vi "NI-USB-6210_Kernel.vi"() -> (0 "error out":errorcluster)   [LabVIEW 2013]
uses:
  <vilib>/DAQmx/read.llb/DAQmx Read (Analog 2D DBL NChan NSamp).vi
  Globals/measurementGlobal.vi
  <vilib>/DAQmx/configure/timing.llb/DAQmx Timing (Sample Clock).vi
  <vilib>/DAQmx/create/channels.llb/DAQmx Create Channel (AI-Voltage-Basic).vi
  <vilib>/DAQmx/miscellaneous.llb/DAQmx Fill In Error Info.vi
panel:
  out "Block Index":i32
  out "Case":string[](array[string])
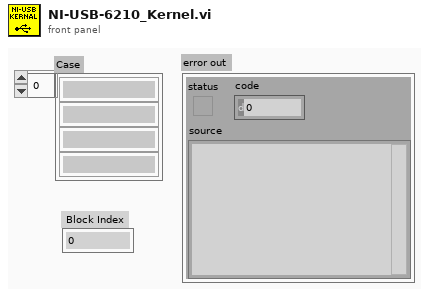
[diagram p1: front panel]
types:
  T1 = cluster{"No of Chans":i32, "Low Volt Limit (-10V)":dbl, "High Volt Limit (10V)":dbl}[]
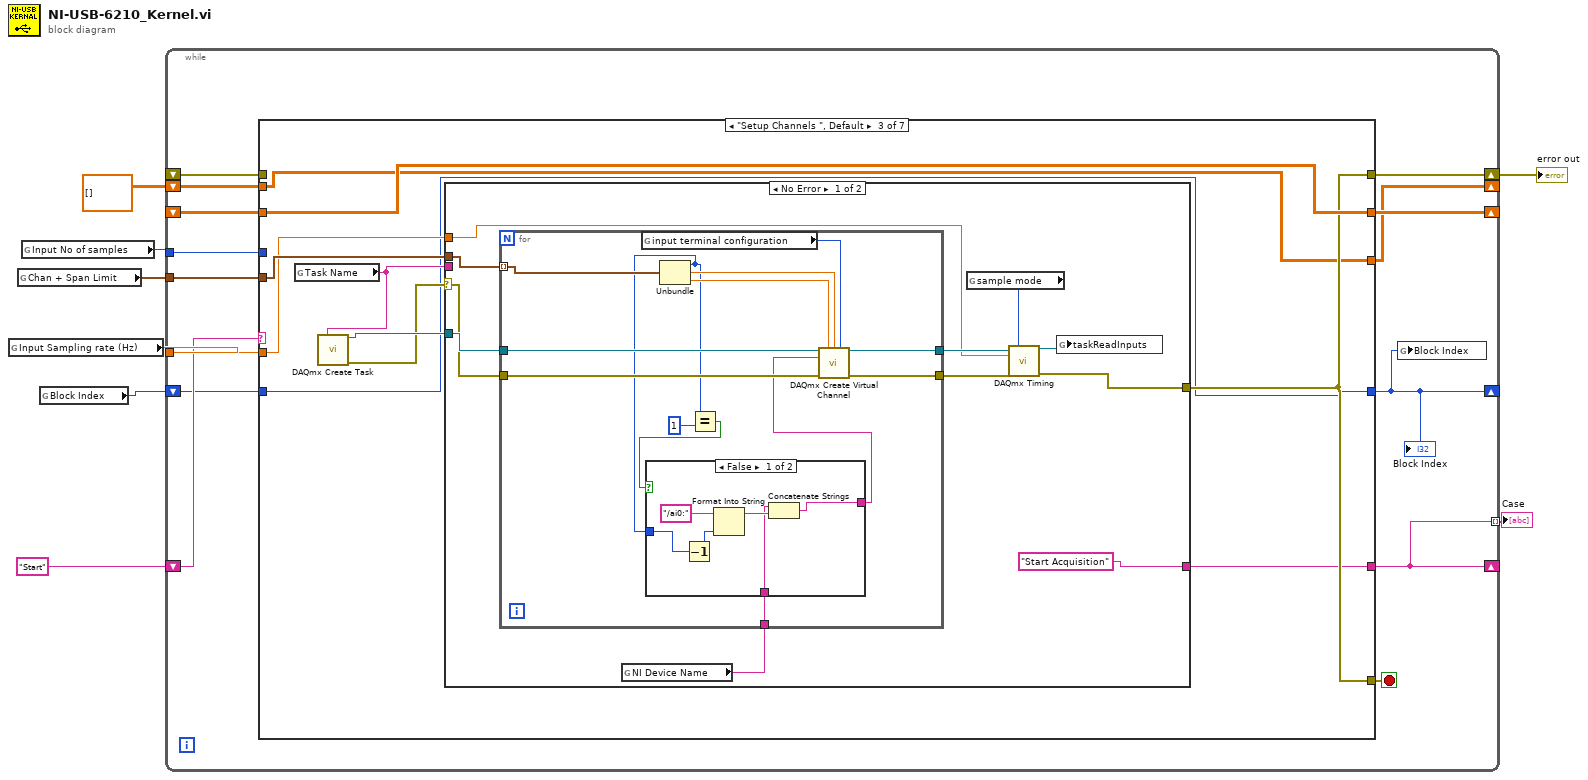
[diagram p0: block diagram]
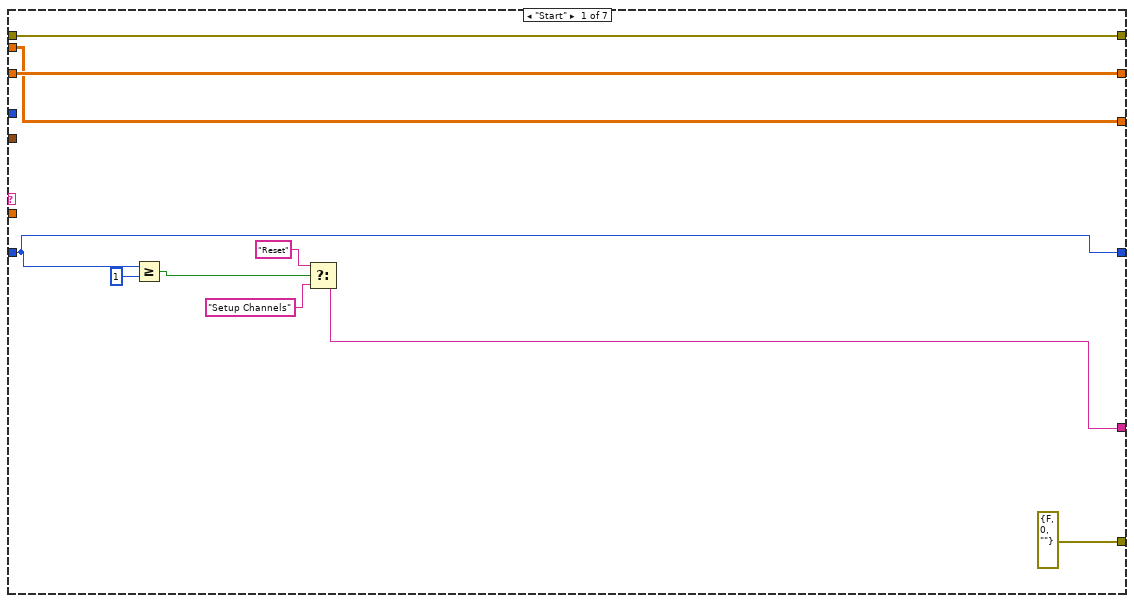
[diagram p2: hidden frame]
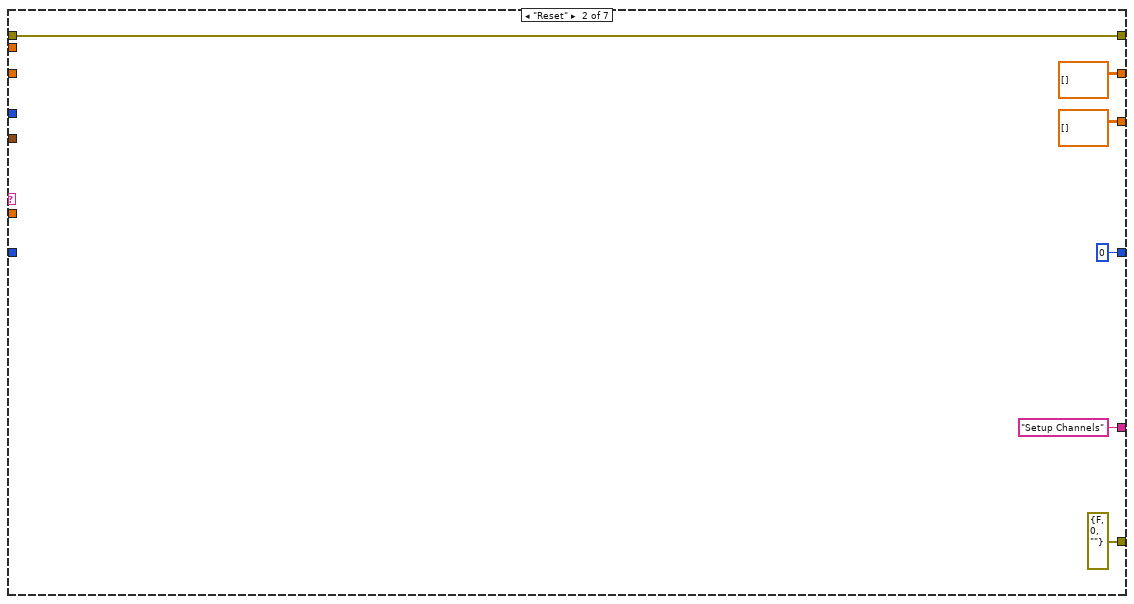
[diagram p3: hidden frame]
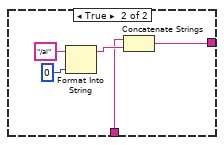
[diagram p4: hidden frame]
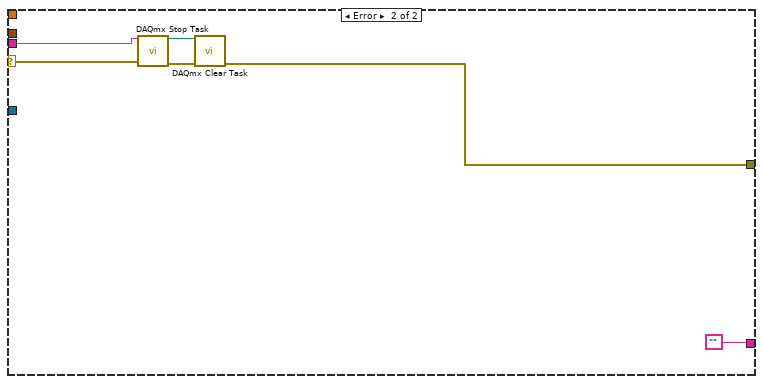
[diagram p5: hidden frame]
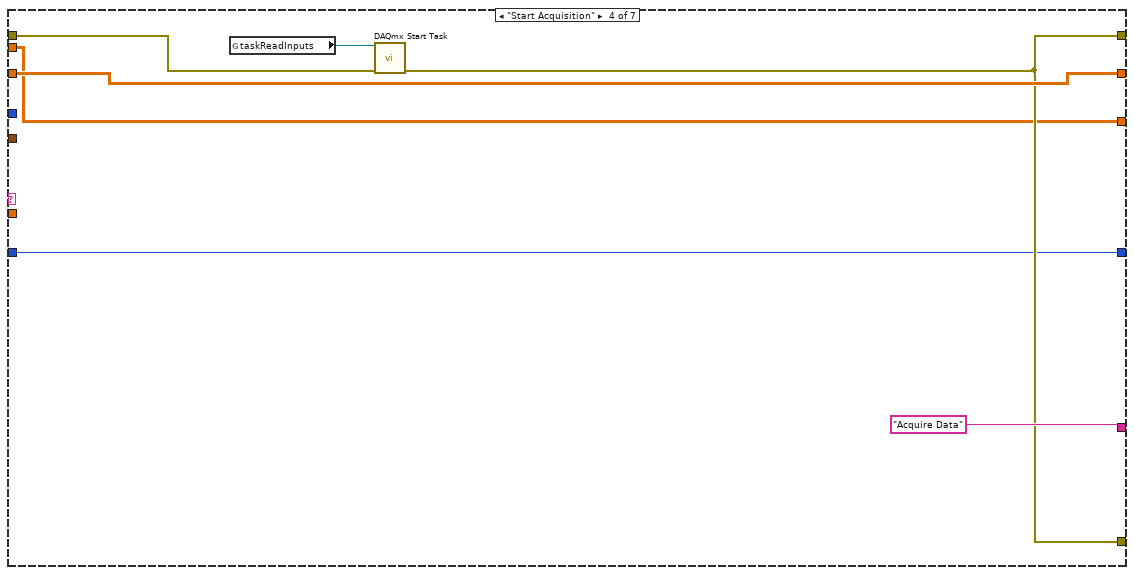
[diagram p6: hidden frame]
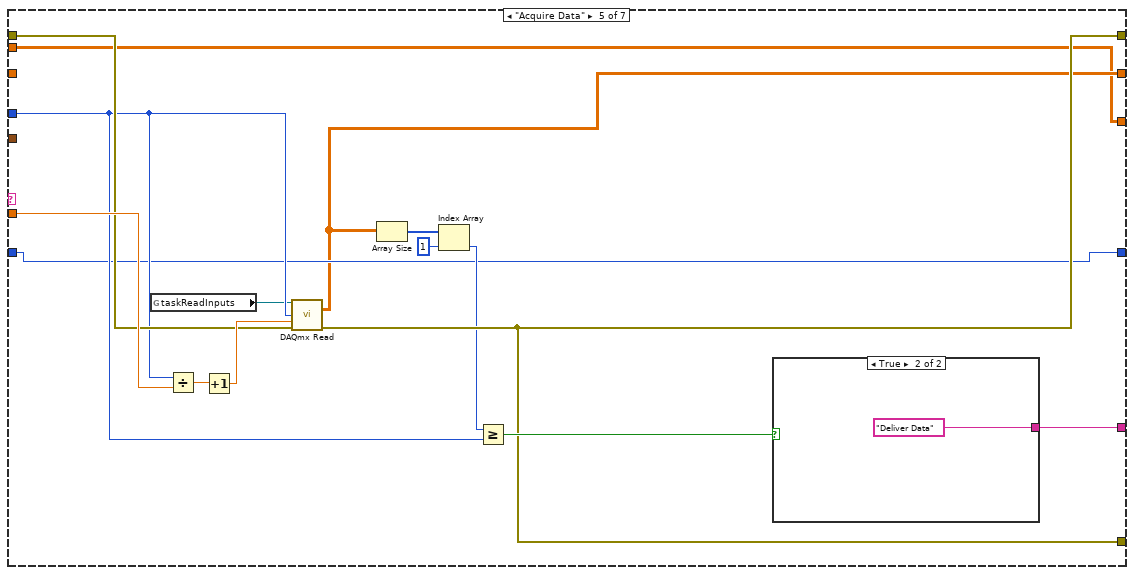
[diagram p7: hidden frame]
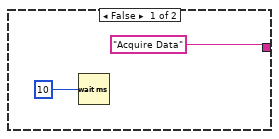
[diagram p8: hidden frame]
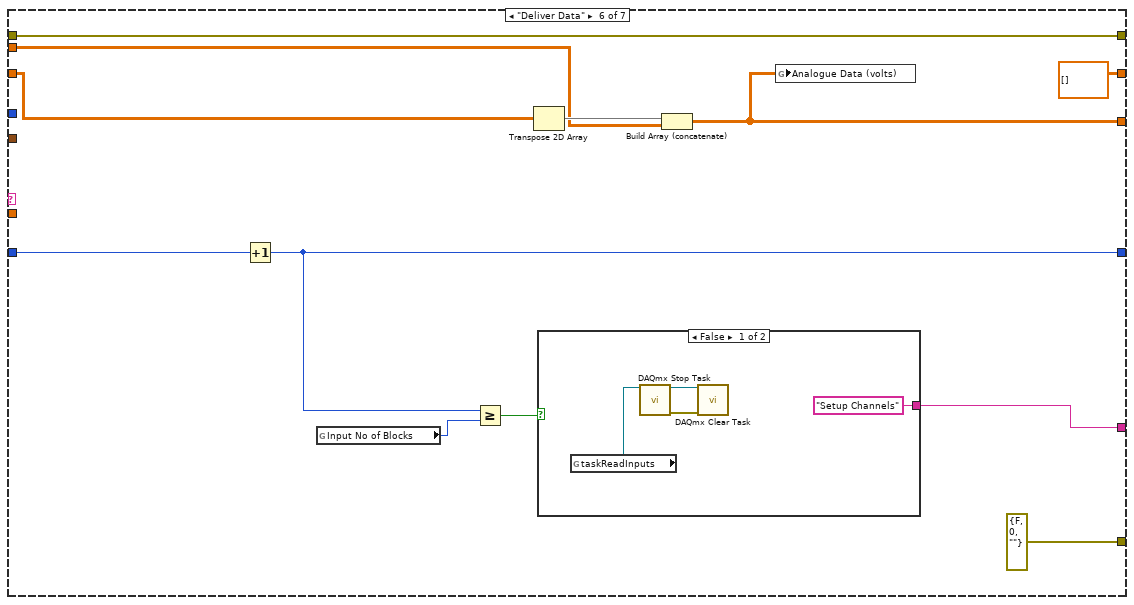
[diagram p9: hidden frame]
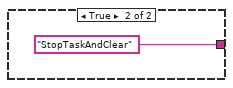
[diagram p10: hidden frame]
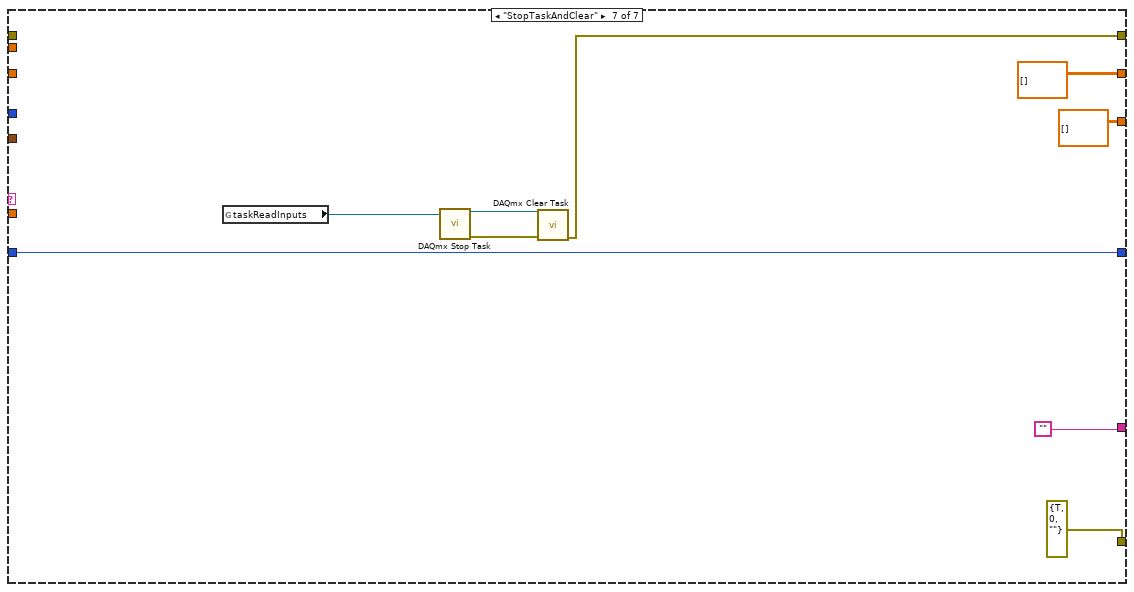
[diagram p11: hidden frame]
diagram:
  n1 = global read "measurementGlobal.vi" "Input Sampling rate (Hz)"() -> (w7:dbl)
  n2 = global read "measurementGlobal.vi" "Chan + Span Limit"() -> (w3:T1)
  n3 = global read "measurementGlobal.vi" "Input No of samples"() -> (w8:i32)
  n4 = global read "measurementGlobal.vi" "Block Index"() -> (w2:i32)
  n5 = while {
    tunnel: w8 -> [w22]
    tunnel: w7 -> [w21]
    shift-right: [w20] -> w6
    shift-left: _ -> [w19]
    shift-right: [w10] -> _
    shift-left: _ -> [w17]
    shift-right: [w15] -> _
    shift-left: "Start" -> [w16]
    tunnel: [w15] -> w4 mode=indexing
    tunnel: w3 -> [w14]
    shift-right: [w12] -> _
    shift-left: w2 -> [w13]
    shift-right: [w9] -> _
    shift-left: dbl[][] [] ("data") -> [w11]
    stop <- w18 stop-if-true
    n6 = case shown="\"Setup Channels \", Default" w16 {
      tunnel: w22 -> [_ _ _ _ w105 _ _]
      tunnel: w21 -> [_ _ w43 _ w111 _ _]
      tunnel: [w25 w35 w42 w92 w102 w126 w138] -> w20
      tunnel: w19 -> [w25 w35 _ w95 w108 w126 _]
      tunnel: [errorcluster {"status"=FALSE, "code"=0, "source"=""} ("error out") errorcluster {"status"=FALSE, "code"=0, "source"=""} ("error out") w42 w92 w102 errorcluster {"status"=FALSE, "code"=0, "source"=""} ("error out") errorcluster {"status"=TRUE, "code"=0, "source"=""} ("error out")] -> w18
      tunnel: [w32 dbl[][] [] ("data") w48 w94 w98 dbl[][] [] ("data") dbl[][] [] ("data")] -> w10
      tunnel: w17 -> [w32 _ w48 w94 _ w118 _]
      tunnel: [w27 "Setup Channels" ("f") w41 "Acquire Data" w103 w123 ""] -> w15
      tunnel: w14 -> [_ _ w44 _ _ _ _]
      tunnel: w13 -> [w26 _ w40 w91 w99 w120 w133]
      tunnel: [w26 0 ("Block Index") w40 w91 w99 w119 w133] -> w12
      tunnel: w11 -> [w23 _ w39 w90 w97 w116 _]
      tunnel: [w23 dbl[][] [] ("data") w39 w90 w97 w115 dbl[][] [] ("data")] -> w9
      frame "Start" {
        n7 = Greater Or Equal?(x=w26, y=1) -> (x >= y?=w30:bool)
        n8 = Select(t="Reset", s=w30, f="Setup Channels") -> (s? t:f=w27:string)
      }
      frame "Reset" {
      }
      frame "Setup Channels ", Default {
        n9 = global read "measurementGlobal.vi" "Task Name"() -> (w45:string)
        n10 = call <vilib>:"DAQmx Create Task.vi"("new task name"=w45) -> ("task out"=w47:refnum<k21>, "error out"=w46:errorcluster)  [unwired: 13 in]
        n11 = case shown="No Error" w46 {
          selector: w46 -> [w57 w86]
          tunnel: w44 -> [w56 _]
          tunnel: w47 -> [w58 _]
          tunnel: w45 -> [_ w88]
          tunnel: [w50 w85] -> w42
          tunnel: w43 -> [w52 _]
          tunnel: ["Start Acquisition" ""] -> w41
          frame No Error {
            n12 = global read "measurementGlobal.vi" "NI Device Name"() -> (w59:string)
            n13 = for {
              tunnel: w56 -> [w72] mode=indexing
              tunnel: w59 -> [w62]
              tunnel: [w69] -> w53
              tunnel: [w68] -> w51
              tunnel: w58 -> [w66]
              tunnel: w57 -> [w65]
              n14 = global read "measurementGlobal.vi" "input terminal configuration"() -> (w67:i32)
              n15 = Unbundle(w72) -> ("No of Chans"=w61:i32, "Low Volt Limit (-10V)"=w71:dbl, "High Volt Limit (10V)"=w70:dbl)
              n16 = Equal?(x=w61, y=1) -> (x = y?=w63:bool)
              n17 = case shown="False" w63 {
                tunnel: w62 -> [w73 w81]
                tunnel: [w76 w80] -> w60
                tunnel: w61 -> [w75 _]
                frame False {
                  n18 = Decrement(x=w75) -> (x-1=w74:i32)
                  n19 = Format Into String(initial string="/ai0:", w74) -> (resulting string=w78:string)  [unwired: 2 in, 1 out]
                  n20 = Concatenate Strings(w73, w78) -> (w76:string)
                }
                frame True {
                  n21 = Format Into String(initial string="/ai", 0 ("input 1")) -> (resulting string=w82:string)  [unwired: 2 in, 1 out]
                  n22 = Concatenate Strings(w81, w82) -> (w80:string)
                }
              }
              n23 = call-poly <vilib>:"DAQmx Create Virtual Channel.vi"("task in"=w66, "maximum value"=w70, "minimum value"=w71, "input terminal configuration"=w67, "physical channels"=w60, "error in"=w65) -> ("task out"=w69:refnum<k21>, "error out"=w68:errorcluster)  [unwired: 8 in]
            }
            n24 = global read "measurementGlobal.vi" "sample mode"() -> (w55:i32)
            n25 = call-poly <vilib>:"DAQmx Timing.vi"("task/channels in"=w53, "sample mode"=w55, "rate"=w52, "error in"=w51) -> ("task out"=w54:refnum<k21>, "error out"=w50:errorcluster)  [unwired: 10 in]
            n26 = global write "measurementGlobal.vi" "taskReadInputs"(w54) -> ()
          }
          frame Error {
            n27 = call <vilib>:"DAQmx Stop Task.vi"("task/channels in"=w88, "error in"=w86) -> ("task out"=w87:refnum<k21>, "error out"=w89:errorcluster)  [unwired: 12 in]
            n28 = call <vilib>:"DAQmx Clear Task.vi"("task in"=w87, "error in"=w89) -> ("error out"=w85:errorcluster)  [unwired: 13 in]
          }
        }
      }
      frame "Start Acquisition" {
        n29 = global read "measurementGlobal.vi" "taskReadInputs"() -> (w96:refnum<k21>)
        n30 = call <vilib>:"DAQmx Start Task.vi"("task/channels in"=w96, "error in"=w95) -> ("error out"=w92:errorcluster)  [unwired: 12 in, 1 out]
      }
      frame "Acquire Data" {
        n31 = global read "measurementGlobal.vi" "taskReadInputs"() -> (w101:refnum<k21>)
        n32 = Divide(x=w105, y=w111) -> (x/y=w110:dbl)
        n33 = Increment(x=w110) -> (x+1=w109:dbl)
        n34 = call-poly <vilib>:"DAQmx Read.vi"("task/channels in"=w101, "number of samples per channel"=w105, "timeout"=w109, "error in"=w108) -> ("data"=w98:dbl[][], "error out"=w102:errorcluster)  [unwired: 9 in, 1 out]
        n35 = Array Size(array=w98) -> (size(s)=w107:i32[])
        n36 = Index Array(array=w107, index=1) -> (element=w100:i32)
        n37 = Greater Or Equal?(x=w100, y=w105) -> (x >= y?=w104:bool)
        n38 = case shown="True" w104 {
          tunnel: ["Acquire Data" "Deliver Data"] -> w103
          frame False {
            n39 = Wait (ms)(milliseconds to wait=u32 10) -> ()  [unwired: 1 out]
          }
          frame True {
          }
        }
      }
      frame "Deliver Data" {
        n40 = Increment(x=w120) -> (x+1=w119:i32)
        n41 = global read "measurementGlobal.vi" "Input No of Blocks"() -> (w125:i32)
        n42 = Greater Or Equal?(x=w119, y=w125) -> (x >= y?=w124:bool)
        n43 = Transpose 2D Array(2D array=w118) -> (transposed array=w117:dbl[][])
        n44 = case shown="False" w124 {
          tunnel: ["Setup Channels" "StopTaskAndClear"] -> w123
          frame False {
            n45 = global read "measurementGlobal.vi" "taskReadInputs"() -> (w128:refnum<k21>)
            n46 = call <vilib>:"DAQmx Stop Task.vi"("task/channels in"=w128) -> ("task out"=w130:refnum<k21>, "error out"=w129:errorcluster)  [unwired: 13 in]
            n47 = call <vilib>:"DAQmx Clear Task.vi"("task in"=w130, "error in"=w129) -> ()  [unwired: 13 in, 1 out]
          }
          frame True {
          }
        }
        n48 = Build Array (concatenate)(w117, w116) -> (w115:dbl[][])
        n49 = global write "measurementGlobal.vi" "Analogue Data (volts)"(w115) -> ()
      }
      frame "StopTaskAndClear" {
        n50 = global read "measurementGlobal.vi" "taskReadInputs"() -> (w140:refnum<k21>)
        n51 = call <vilib>:"DAQmx Stop Task.vi"("task/channels in"=w140) -> ("task out"=w137:refnum<k21>, "error out"=w139:errorcluster)  [unwired: 13 in]
        n52 = call <vilib>:"DAQmx Clear Task.vi"("task in"=w137, "error in"=w139) -> ("error out"=w138:errorcluster)  [unwired: 13 in]
      }
    }
    "Block Index" <- w12
    n53 = global write "measurementGlobal.vi" "Block Index"(w12) -> ()
  }
  "error out" <- w6
  "Case" <- w4
